vi "startHW.vi"(8 "error in (no error)":errorcluster, 11 "WindowsTarget in":refnum<class "WindowsTarget.lvclass">) -> (0 "error out":errorcluster, 3 "WindowsTarget out":refnum<class "WindowsTarget.lvclass">)   [LabVIEW 2012, in "WindowsTarget.lvclass"]
doc: "Performs any operations necessary to start the hardware. This Windows version generates a user event with the loop time for use elsewhere."
uses:
  WindowsTarget.lvclass
  WindowsTarget.lvclass/WindowsTarget.ctl
  C/Program Files (x86)/National Instruments/LabVIEW 2012/user.lib/Common/ComponentModel/ComponentModelRT/LoopTimer/ILoopTimer/ILoopTimer.lvclass
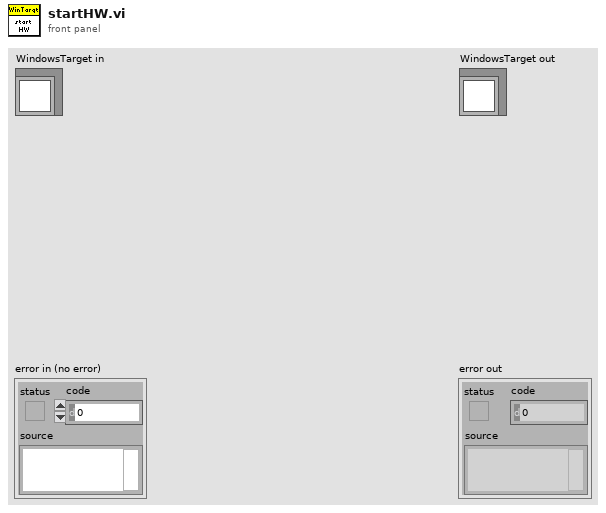
[diagram p1: front panel]
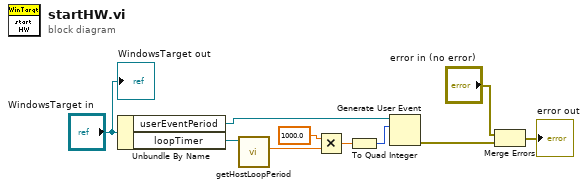
[diagram p0: block diagram]
diagram:
  n1 = Unbundle By Name("WindowsTarget in") -> ("userEventPeriod"=w10:refnum<user-event>, "loopTimer"=w7:refnum<class "ILoopTimer.lvclass">)
  n2 = call-dynamic "getHostLoopPeriod.vi"("ILoopTimer in"=w7) -> ("hostLoopPeriod_s"=w5:dbl)  [unwired: 8 in, 2 out]
  n3 = Multiply(x=1000.0 ("y"), y=w5) -> (x*y=w9:dbl)
  n4 = To Quad Integer(1:w9) -> (0:w8:i64)
  n5 = Generate User Event(user event=w10, event data cluster=w8) -> (error out=w2:errorcluster)  [unwired: 1 in, 1 out]
  n6 = Merge Errors("error in (no error)", w2) -> (→"error out":errorcluster)
  "WindowsTarget out" <- "WindowsTarget in"
